vi "NicmosCloseSynchronization.vi"(2 "Synchronization":T1, 9 "error out":errorcluster caption="error in (no error)") -> (6 "error in (no error)":errorcluster caption="error out")   [LabVIEW 2009]
uses:
  Controls/NicmosSynchronization.ctl
  Controls/NICMOS.COMMAND.QUEUE.ctl
  Controls/NICMOS.COMMAND.ctl
  Controls/NICMOS.COMMANDBASIC.ctl
  Controls/NICMOS.READOUT.ctl
  Controls/NICMOS.FILTERCOMMAND.ctl
  Controls/NICMOS.FILTER.ctl
  Controls/NICMOS.STATE.NOTIFIER.ctl
  Controls/NICMOS.STATE.ctl
  Controls/NICMOS.DATA.NOTIFIER.ctl
  Controls/NICMOS.DATA.ctl
  Controls/NICMOS.DATA.QUEUE.ctl
  Controls/NICMOS.RAW.NOTIFIER.ctl
  Controls/NICMOS.RAW.ctl
  Controls/NICMOS.TEMPERATURE.NOTIFIER.ctl
  Controls/NICMOS.TEMPERATURE.ctl
  Controls/NICMOS.READOUT.NOTIFIER.ctl
  Controls/NICMOS.FILTER.NOTIFIER.ctl
  Controls/NICMOS.MASKBANKS.NOTIFIER.ctl
  Controls/NICMOS.MASKBANKS.ctl
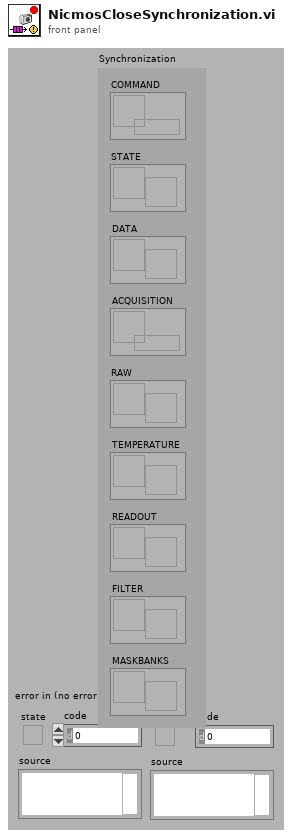
[diagram p1: front panel]
types:
  T1 = typedef "NicmosSynchronization.ctl" = cluster{"COMMAND":T2, "STATE":T3, "DATA":T4, "ACQUISITION":T5, "RAW":T6, "TEMPERATURE":T7, "READOUT":T8, "FILTER":T9, "MASKBANKS":T10}
  T2 = typedef "NICMOS.COMMAND.QUEUE.ctl" = refnum<queue>
  T3 = typedef "NICMOS.STATE.NOTIFIER.ctl" = refnum<notifier>
  T4 = typedef "NICMOS.DATA.NOTIFIER.ctl" = refnum<notifier>
  T5 = typedef "NICMOS.DATA.QUEUE.ctl" = refnum<queue>
  T6 = typedef "NICMOS.RAW.NOTIFIER.ctl" = refnum<notifier>
  T7 = typedef "NICMOS.TEMPERATURE.NOTIFIER.ctl" = refnum<notifier>
  T8 = typedef "NICMOS.READOUT.NOTIFIER.ctl" = refnum<notifier>
  T9 = typedef "NICMOS.FILTER.NOTIFIER.ctl" = refnum<notifier>
  T10 = typedef "NICMOS.MASKBANKS.NOTIFIER.ctl" = refnum<notifier>
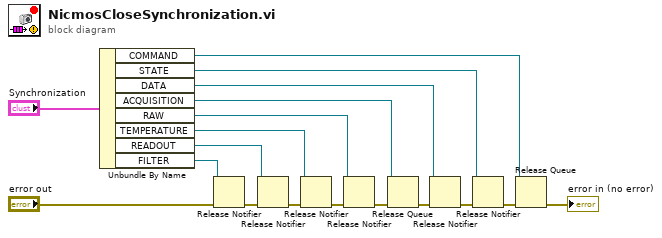
[diagram p0: block diagram]
diagram:
  n1 = Unbundle By Name("Synchronization") -> ("COMMAND"=w12:T2, "STATE"=w13:T3, "DATA"=w14:T4, "ACQUISITION"=w1:T5, "RAW"=w15:T6, "TEMPERATURE"=w16:T7, "READOUT"=w17:T8, "FILTER"=w5:T9)
  n2 = Release Notifier(notifier=w5, error in (no error)="error out") -> (error out=w6:errorcluster)  [unwired: 1 in, 2 out]
  n3 = Release Notifier(notifier=w17, error in (no error)=w6) -> (error out=w10:errorcluster)  [unwired: 1 in, 2 out]
  n4 = Release Notifier(notifier=w16, error in (no error)=w10) -> (error out=w9:errorcluster)  [unwired: 1 in, 2 out]
  n5 = Release Notifier(notifier=w15, error in (no error)=w9) -> (error out=w3:errorcluster)  [unwired: 1 in, 2 out]
  n6 = Release Queue(queue=w1, error in (no error)=w3) -> (error out=w2:errorcluster)  [unwired: 1 in, 2 out]
  n7 = Release Notifier(notifier=w14, error in (no error)=w2) -> (error out=w8:errorcluster)  [unwired: 1 in, 2 out]
  n8 = Release Notifier(notifier=w13, error in (no error)=w8) -> (error out=w7:errorcluster)  [unwired: 1 in, 2 out]
  n9 = Release Queue(queue=w12, error in (no error)=w7) -> (error out=→"error in (no error)":errorcluster)  [unwired: 1 in, 2 out]
